vi "Insight Int Package.vi"(2 "Footer":string, 3 "Int32":i32, 4 "Header":string) -> (0 "resulting string":string)   [LabVIEW 2013]
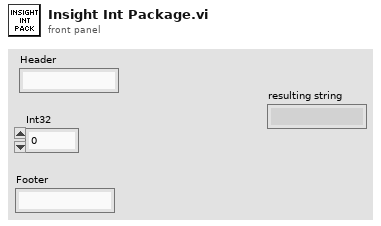
[diagram p1: front panel]
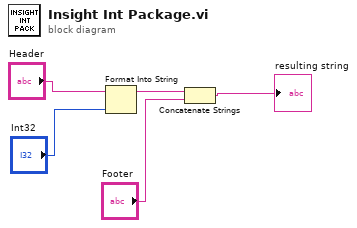
[diagram p0: block diagram]
diagram:
  n1 = Format Into String(initial string="Header", "Int32") -> (resulting string=w1:string)  [unwired: 2 in, 1 out]
  n2 = Concatenate Strings(w1, "Footer") -> (→"resulting string":string)
